vi "Remove Duplicate Points.vi"(8 "error in (no error)":errorcluster, 11 "Tool Object in":refnum<class "Tool Object.lvclass">) -> (0 "error out":errorcluster, 3 "Tool Object out":refnum<class "Tool Object.lvclass">)   [LabVIEW 2019, in "Tool Object.lvclass"]
uses:
  Tool Object.lvclass
  Parse/PathCommands/Point.ctl
  Parse/PathCommands/PathCommands.lvclass
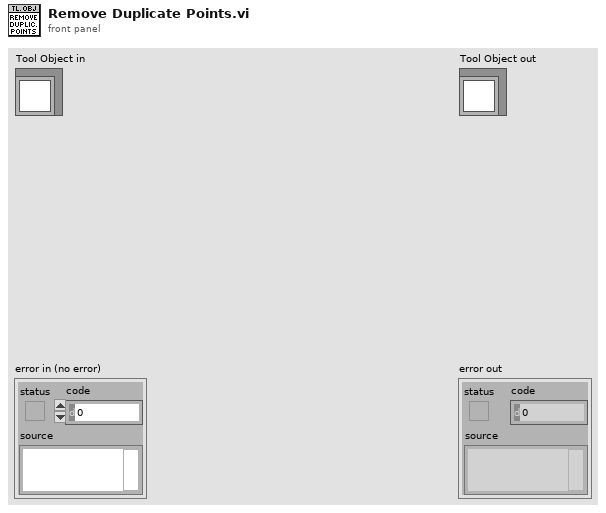
[diagram p1: front panel]
types:
  T1 = typedef "PathCommands.lvclass/Point.ctl" = cluster{"X":dbl, "Y":dbl}
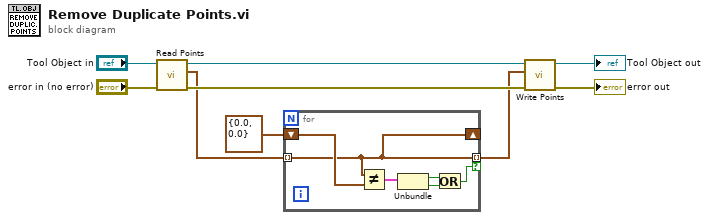
[diagram p0: block diagram]
diagram:
  n1 = call-dynamic "Read Points.vi"("error in (no error)"="error in (no error)", "Tool Object in"="Tool Object in") -> ("error out"=w5:errorcluster, "Points"=w2:T1[], "Tool Object out"=w8:refnum<class "Tool Object.lvclass">)  [unwired: 7 in]
  n2 = for {
    tunnel: w2 -> [w14] mode=indexing
    tunnel: [w14] -> w1 mode=indexing if=w10
    shift-right: [w14] -> _
    shift-left: T1 {"X"=0.0, "Y"=0.0} ("Point") -> [w15]
    n3 = Not Equal?(x=w14, y=w15) -> (x != y?=w13:cluster{"X":bool, "Y":bool})
    n4 = Unbundle(w13) -> ("X"=w12:bool, "Y"=w11:bool)
    n5 = Or(x=w12, y=w11) -> (x .or. y?=w10:bool)
  }
  n6 = call-dynamic "Write Points.vi"("error in (no error)"=w5, "Points"=w1, "Tool Object in"=w8) -> ("error out"=→"error out":errorcluster, "Tool Object out"=→"Tool Object out":refnum<class "Tool Object.lvclass">)  [unwired: 7 in]
